vi "GetFileMethod.vi"(0 "object in":refnum<class "Client.lvclass">, 5 "Error In":errorcluster) -> (14 "object out":refnum<class "Client.lvclass">, 15 "File Method":T1, 19 "Error Out":errorcluster)   [LabVIEW 2024, in "Client.lvclass"]
uses:
  <resource>/Framework/Providers/Open_GDS/ClassProviders/Provider_LvNativeClass/Templates/NativeBaseTemplate/NativeBaseTemplate.lvclass/NativeBaseTemplate.ctl
  Client.lvclass
  Client.lvclass/Client.ctl
  Support/Type Def/File Method.ctl
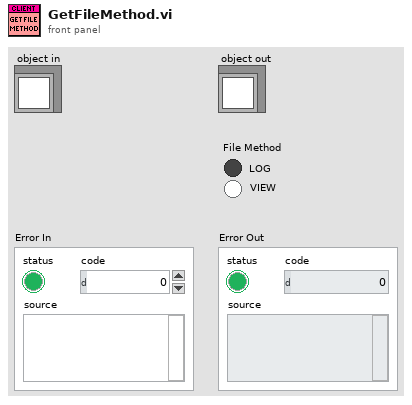
[diagram p1: front panel]
types:
  T1 = typedef "File Method.ctl" = enum32{"Log", "View"}
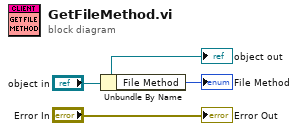
[diagram p0: block diagram]
diagram:
  n1 = Unbundle By Name("object in") -> ("File Method"=→"File Method":T1)
  "Error Out" <- "Error In"
  "object out" <- "object in"
